vi "User-Defined IO Variable - Basic (Host) - PXI.vi"() -> ()   [LabVIEW 2015]
doc: "This VI shows how to pass values from the host to the FPGA and back from the FPGA to the host using the user-defined I/O variable. It also shows how to use user-defined I/O variable scaling."
uses:
  <vilib>/Platform/TimedLoop/XDataNode/timing_clust.ctl
  <vilib>/Platform/TimedLoop/XDataNode/nitl_modes.ctl
  <vilib>/Platform/TimedLoop/XDataNode/wakeup.ctl
  <vilib>/platform/TimedLoop/XDataNode/XDataNode.xnode
  <vilib>/Platform/TimedLoop/XDataNode/XDNodeRunTimeDep.lvlib
panel:
  out "Waveform Chart":cluster{i16, i16}(graph)
  in  "HF: Boolean":bool
  in  "HF: Int":u32
  out "FPGA to Host: Boolean":bool
  in  "Stop":bool
  out "FPGA to Host: Integer":u32
  # "Overview: Demonstrates how to pass values to and from the FPGA through user-defined I/O variables. Refer to the Transferring Data Between the FPGA and Host VI (FPGA Module) topic of the LabVIEW Help for more information.\nRequirements: LabVIEW Real-Time Module, LabVIEW FPGA Module, NI-RIO\nInstructions: \n1. Compile the FPGA VI\n2. Run the VI.\n3. Enter a value, from 0-10, in the Host to FPGA: Integer control. The FPGA to Host: Integer indicator will return the value scaled to a range of 0-100. The scaling can be configured in the User-Defined I/O Variable properties page, accessible from the project.\n4. Click Stop to stop the VI."
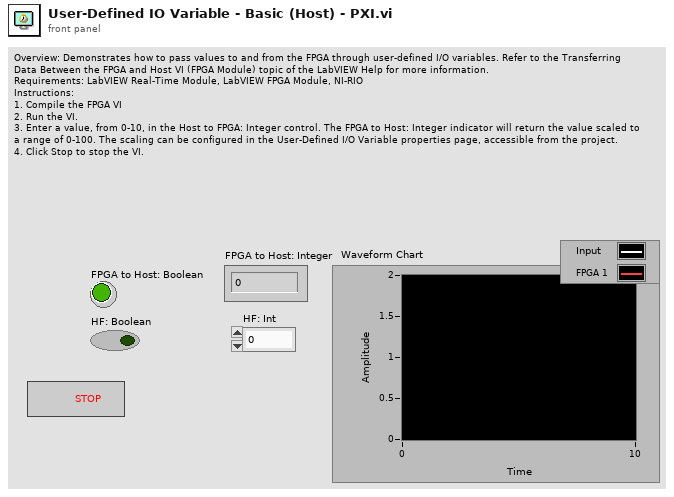
[diagram p1: front panel]
types:
  T1 = typedef "XDNodeRunTimeDep.lvlib/timing_clust.ctl" = cluster{"Expected End [f-1]":u64, "Actual End [f-1]":u64, "Finished Late? [f-1]":bool, "Expected End [i-1]":u64, "Actual End [i-1]":u64, "Finished Late? [i-1]":bool, "Expected Start [i]":u64, "Actual Start [i]":u64, "Expected Start [f]":u64, "Actual Start [f]":u64, "Source Name":string, "Structure Name":string, "Period":i64, "Deadline":i64, "Offset":i64, "Start":i64, "Priority":i32, "Timeout":i32, "Mode":T2, "Wakeup Reason":T3, "Error":errorcluster, "Source Type":string, "Secondary Source Type":string, "Global End Time":u64, "Global Start Time":u64, "Frame Duration":u64, "Iteration Duration":u64, "Assigned CPU":i32, "I/O Scan Engine Mode":u32}
  T2 = typedef "XDNodeRunTimeDep.lvlib/nitl_modes.ctl" = enum32{"No Change", "Process missed periods, maintain original phase", "Discard missed periods, maintain original phase", "Process missed periods, ignore original phase", "Discard missed periods, ignore original phase"}
  T3 = typedef "XDNodeRunTimeDep.lvlib/wakeup.ctl" = enum32{"Normal", "Aborted", "Asynchronous wakeup", "Timing source error", "Timed loop error", "Timeout"}
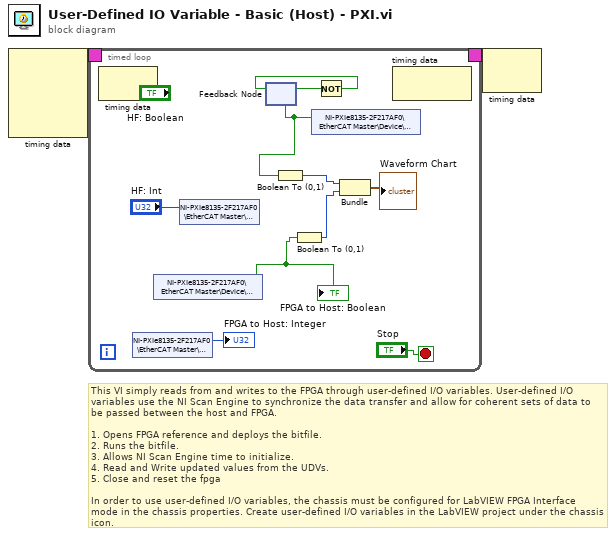
[diagram p0: block diagram]
diagram:
  # "This VI simply reads from and writes to the FPGA through user-defined I/O variables. User-defined I/O variables use the NI Scan Engine to synchronize the data transfer and allow for coherent sets of data to be passed between the host and FPGA. \n\n1. Opens FPGA reference and deploys the bitfile.\n2. Runs the bitfile.\n3. Allows NI Scan Engine time to initialize.\n4. Read and Write updated values from the UDVs. \n5. Close and reset the fpga\n\nIn order to use user-defined I/O variables, the chassis must be configured for LabVIEW FPGA Interface mode in the chassis properties. Create user-defined I/O variables in the LabVIEW project under the chassis icon."
  n1 = node-c288() -> (w2:T1)  [unwired: 4 in]
  n2 = timed-loop {
    timing: w2 -> [_]
    timing-out: [_] -> w1
    stop <- "Stop" stop-if-true
    n3 = node-c288() -> ()  [unwired: 1 in, 1 out]
    n4 = shared-variable "NI-PXIe8135-2F217AF0\\EtherCAT Master\\Device\\User-Defined Variables\\FH: Int"() -> (→"FPGA to Host: Integer":u32)  [unwired: 1 in, 1 out]
    n5 = shared-variable "NI-PXIe8135-2F217AF0\\EtherCAT Master\\Device\\User-Defined Variables\\FH: Boolean"() -> (w7:bool)  [unwired: 1 in, 1 out]
    "FPGA to Host: Boolean" <- w7
    n6 = shared-variable "NI-PXIe8135-2F217AF0\\EtherCAT Master\\Device\\User-Defined Variables\\HF: Int"("HF: Int") -> ()  [unwired: 1 in, 1 out]
    n7 = feedback #1() -> (w6:bool)  [unwired: 1 in]
    n8 = Boolean To (0,1)(Boolean=w6) -> (0, 1=w4:i16)
    n9 = Boolean To (0,1)(Boolean=w7) -> (0, 1=w3:i16)
    n10 = shared-variable "NI-PXIe8135-2F217AF0\\EtherCAT Master\\Device\\User-Defined Variables\\HF: Boolean"(w6) -> ()  [unwired: 1 in, 1 out]
    n11 = Not(x=w6) -> (.not. x?=w8:bool)
    n12 = feedback-in #1(w8) -> ()
    n13 = Bundle(w4, w3) -> (→"Waveform Chart":cluster{i16, i16})  [unwired: 1 out]
    n14 = node-c288() -> ()  [unwired: 1 in, 1 out]
  }
  n15 = node-c288(w1) -> ()  [unwired: 1 out]
